vi "SA_OpenSystem.vi"(8 "error in (no error)":errorcluster, 10 "options":string, 11 "systemLocator":string) -> (0 "error out":errorcluster, 3 "systemIndexOut":u32)   [LabVIEW 2013]
doc: "<B>Description:</B>\nThis function initializes one MCS. The communication mode (synchronous or asynchronous) can be configured.\n<B>Parameters:</B>\n<B>- systemLocator</B> (string), input - The system locator describes the communication interface and the location of a MCS device. Depending on the interface type the format of the locator varies:\nUSB Interfaces: The locator format is <B>usb:id:123456789</B> where 123456789 is the system ID which is the first part of the device serial number (usually printed on the backside of the MCS). The format <B>usb:ix:0</B> can be used to address the nth device in the list of connected MCS/USB. This method is not recommended, because the order of connected USB devices can change between sessions.\nNetwork Interfaces: The locator format is <B>network:192.168.1.200:5000</B> where 192.168.1.200 is the IP address and 5000 the port of the MCS. Since IP adress and port can be configured for a MCS/Network device, the correct IP and port may be different.\n<B>- options</B> (string), input - Use this parameter to pass options to the open command. Multiple options must be separated by a comma or a newline. Possible options are \n - sync: the system is initialize for synchronous communication\n - async: the system is initialized for asynchronous communication\n - reset: the system is reset on open\n<B>- systemIndexOut</B> (unsigned 32bit), output - The system index for the opened system."
uses:
  MCSControl.dll
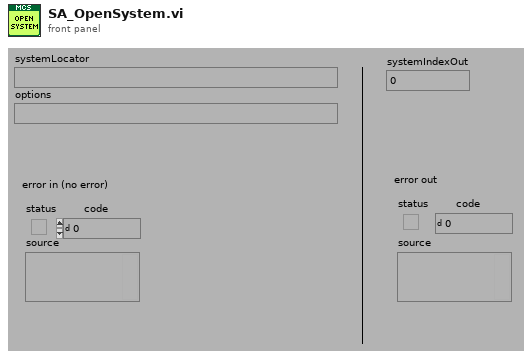
[diagram p1: front panel]
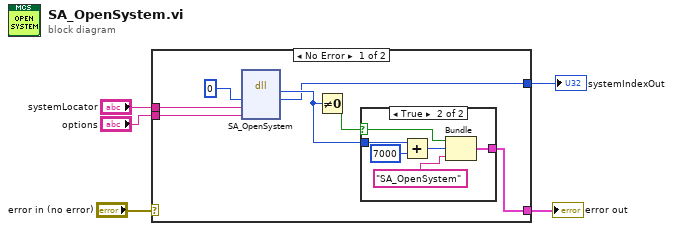
[diagram p0: block diagram]
diagram:
  n1 = case shown="No Error" "error in (no error)" {
    selector: "error in (no error)" -> [_ w19]
    tunnel: [w10 w19] -> w4
    tunnel: "options" -> [w9 _]
    tunnel: "systemLocator" -> [w8 _]
    tunnel: [w6 _] -> w1
    frame No Error {
      n2 = dll-call lib="MCSControl.dll" fn="SA_OpenSystem"("systemIndexOut"=u32 0, "systemLocator"=w8, "options"=w9) -> ("return type"=w11:u32, "systemIndexOut"=w6:u32)  [unwired: 5 in, 2 out]
      n3 = Not Equal To 0?(x=w11) -> (x != 0?=w12:bool)
      n4 = case shown="True" w12 {
        selector: w12 -> [_ w15]
        tunnel: w11 -> [_ w18]
        tunnel: [_ w13] -> w10
        frame False {
        }
        frame True {
          n5 = Add(x=w18, y=u32 7000) -> (x+y=w16:u32)
          n6 = Bundle(w15, w16, "source"="SA_OpenSystem") -> (w13:cluster{bool, u32, "source":string})  [unwired: 1 in]
        }
      }
    }
    frame Error {
    }
  }
  "error out" <- w4
  "systemIndexOut" <- w1
